vi "CM-TDT-Register Events.vi"(10 "List Refs":refnum<vi>[](array[refnum]), 11 "Table Refs":refnum<vi>[](array[refnum])) -> (1 "Lists":cluster{"AO":T2, "AI":T2, "DO":T2, "DI":T2}, 2 "Tables":cluster{"AO":T1, "AI":T1, "DO":T1, "DI":T1}, 3 "Event Registration Refnum":refnum<event-registration>)   [LabVIEW 2020]
uses:
  Utility VIs/Controls/KListboxEx/KListboxEx.xctl
  Utility VIs/Controls/KTable/KTable.xctl
  Utility VIs/Controls/KListboxEx/Events.ctl
  Utility VIs/Controls/KListboxEx/Event Action.ctl
  Utility VIs/Controls/KTable/Events.ctl
  Utility VIs/Controls/KTable/Event Data.ctl
  Utility VIs/Controls/KTable/Event Type.ctl
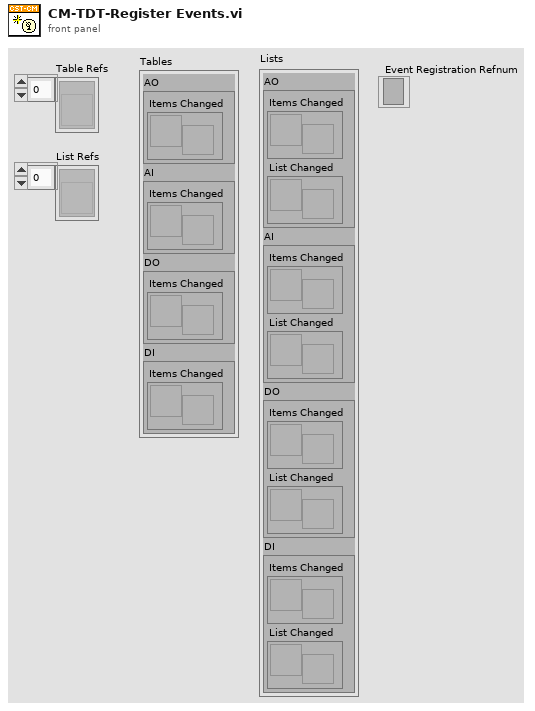
[diagram p1: front panel]
types:
  T1 = typedef "KTable.xctl/Events.ctl" = cluster{"Items Changed":refnum<user-event>}
  T2 = typedef "KListboxEx.xctl/Events.ctl" = cluster{"Items Changed":refnum<user-event>, "List Changed":refnum<user-event>}
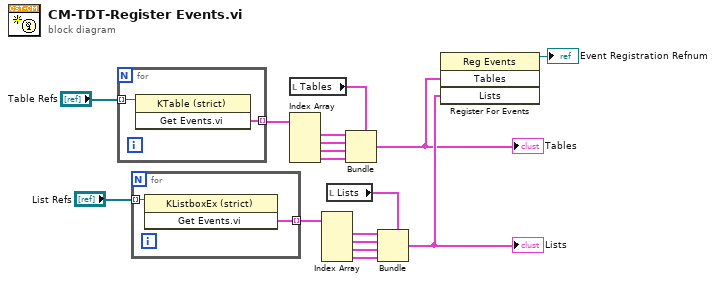
[diagram p0: block diagram]
diagram:
  n1 = for {
    tunnel: "Table Refs" -> [w19] mode=indexing
    tunnel: [w18] -> w4 mode=indexing
    n2 = invoke class="KTable (strict)" method="Get Events.vi"(reference=w19) -> ("Get Events.vi"=w18:T1)  [unwired: 2 in, 2 out]
  }
  n3 = for {
    tunnel: "List Refs" -> [w21] mode=indexing
    tunnel: [w20] -> w14 mode=indexing
    n4 = invoke class="KListboxEx (strict)" method="Get Events.vi"(reference=w21) -> ("Get Events.vi"=w20:T2)  [unwired: 2 in, 2 out]
  }
  n5 = local read "Tables"() -> (w3:cluster{"AO":T1, "AI":T1, "DO":T1, "DI":T1})
  n6 = Index Array(array=w4) -> (element #1=w8:T1, element #2=w7:T1, element #3=w6:T1, element #4=w5:T1)  [unwired: 4 in]
  n7 = Index Array(array=w14) -> (element #1=w13:T2, element #2=w12:T2, element #3=w11:T2, element #4=w10:T2)  [unwired: 4 in]
  n8 = local read "Lists"() -> (w15:cluster{"AO":T2, "AI":T2, "DO":T2, "DI":T2})
  n9 = Bundle(cluster=w3, "AO"=w8, "AI"=w7, "DO"=w6, "DI"=w5) -> (w2:cluster{"AO":T1, "AI":T1, "DO":T1, "DI":T1})
  "Tables" <- w2
  n10 = Bundle(cluster=w15, "AO"=w13, "AI"=w12, "DO"=w11, "DI"=w10) -> (w9:cluster{"AO":T2, "AI":T2, "DO":T2, "DI":T2})
  "Lists" <- w9
  n11 = register-events(w2, w9) -> (reference out=→"Event Registration Refnum":refnum<event-registration>)  [unwired: 2 in, 1 out]
